vi "ResetField.vi"(8 "error in (no error)":errorcluster, 10 "Coordinate":cluster{"x":i16, "y":i16}, 11 "SnakeGame in":refnum<class "SnakeGame.lvclass">) -> (0 "error out":errorcluster, 3 "SnakeGame out":refnum<class "SnakeGame.lvclass">)   [LabVIEW 2019, in "RT_Game.lvlib" / "SnakeGame.lvclass"]
uses:
  SnakeGame.lvclass
  SnakeGame.lvclass/SnakeGame.ctl
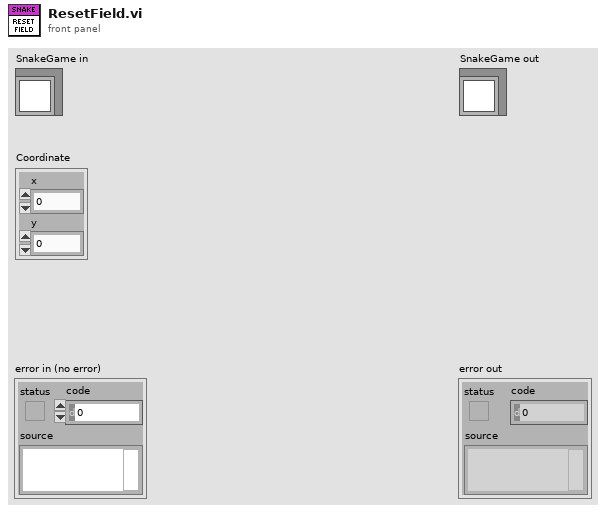
[diagram p1: front panel]
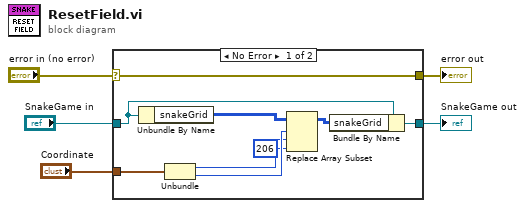
[diagram p0: block diagram]
diagram:
  n1 = case shown="No Error" "error in (no error)" {
    selector: "error in (no error)" -> [w14 w16]
    tunnel: [w14 w16] -> w4
    tunnel: [w11 w15] -> w2
    tunnel: "SnakeGame in" -> [w13 w15]
    tunnel: "Coordinate" -> [w12 _]
    frame No Error {
      n2 = Unbundle By Name(w13) -> ("snakeGrid"=w10:u32[][])
      n3 = Unbundle(w12) -> ("x"=w7:i16, "y"=w8:i16)
      n4 = Replace Array Subset(array=w10, new element=u32 206 ("new element/subarray"), index (row)=w8, index (col)=w7) -> (w9:u32[][])
      n5 = Bundle By Name(cluster=w13, "snakeGrid"=w9) -> (w11:refnum<class "SnakeGame.lvclass">)
    }
    frame Error {
    }
  }
  "error out" <- w4
  "SnakeGame out" <- w2
